vi "Define PDE Domain.vi"   [LabVIEW 2020, in "NI_PDE.lvlib"]
doc: "Defines the domain where you solve the partial differential equation. You must manually select the polymorphic instance to use."
uses:
  <vilib>/gmath/NI_PDE.lvlib
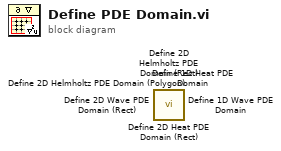
[diagram p0: block diagram]
diagram:
  n1 = call <vilib>:"Define 2D Heat PDE Domain (Rect).vi"() -> ()  [unwired: 14 in, 2 out]
  n2 = call <vilib>:"Define 1D Heat PDE Domain.vi"() -> ()  [unwired: 14 in, 2 out]
  n3 = call <vilib>:"Define 2D Wave PDE Domain (Rect).vi"() -> ()  [unwired: 14 in, 2 out]
  n4 = call <vilib>:"Define 1D Wave PDE Domain.vi"() -> ()  [unwired: 14 in, 2 out]
  n5 = call <vilib>:"Define 2D Helmholtz PDE Domain (Polygon).vi"() -> ()  [unwired: 14 in, 2 out]
  n6 = call <vilib>:"Define 2D Helmholtz PDE Domain (Rect).vi"() -> ()  [unwired: 14 in, 2 out]
